vi "CreateGUID.vi"(8 "error in (no error)":errorcluster) -> (0 "error out":errorcluster, 3 "GUID":string)   [LabVIEW 2015]
uses:
  ole32.dll
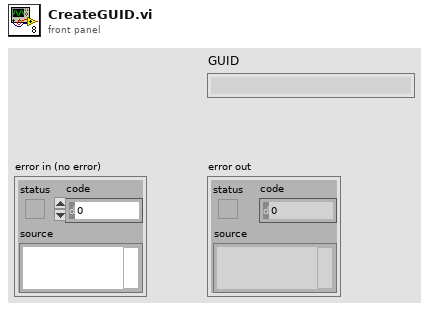
[diagram p1: front panel]
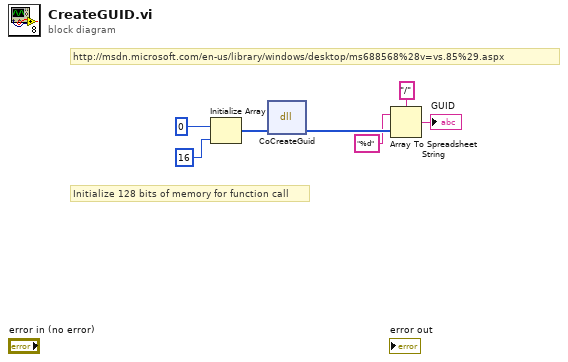
[diagram p0: block diagram]
diagram:
  # "http://msdn.microsoft.com/en-us/library/windows/desktop/ms688568%28v=vs.85%29.aspx"
  # "Initialize 128 bits of memory for function call"
  n1 = Initialize Array(u8 0 ("element"), 16 ("dimension size")) -> (w5:u8[])
  n2 = dll-call lib="ole32.dll" fn="CoCreateGuid"("GUID"=w5) -> ("GUID"=w4:u8[])  [unwired: 4 in, 2 out]
  n3 = Array To Spreadsheet String(delimiter (Tab)="/", array=w4, 3:"%d" ("format string")) -> (spreadsheet string=→"GUID":string)
